vi "Windows Message Queue Example.vi"() -> ()   [LabVIEW 2017, in "Windows messages for Labview (32 and 64).lvlib"]
doc: "This VI demonstrates the use of the Windows Message Queue,\nwhich allows for VIs to be sensitized to specified Windows\nMessages so that they can programmatically respond to the\nmessage.\n\n The call to Create Windows Message Queue configures this VI\nto receive mouse move, left button down and right button down\nmessages. The Wait for Windows Messages waits for the next\nmessage asynchronously. Upon its receipt, it sends all messages\ncurrently in the queue to the case structure that processes them.\n\nIf the Wait times out, we also remove all messages from the\nqueue. This is to prevent messages from building up in the\nqueue when they are not immediately handled. It ensures that\nall messages are processed as soon as possible. \nIt also ensures that if no further messages are received, we still\nprocess the ones currently in the queue after timing out on \nthe Wait.\n\nIf the user clicks in \"Click here to Exit,\" the while loop exits and\nthe Windows message queue is destroyed."
uses:
  Windows messages for Labview (32 and 64).lvlib
  user32.dll
  shell32.dll
panel:
  out "output cluster":cluster{i16, i16}
  out "wParam":u64 format="%.0x"
  out "Files":string[](array[string])
  # "This VI demonstrates the use of the Windows Message Queue,\nwhich allows for VIs to be sensitized to specified Windows\nMessages so that they can programmatically respond to the\nmessage.\n\n The call to Create Windows Message Queue configures this VI\nto receive mouse move, left button down and right button down\nmessages.  The Wait for Windows Messages waits for the next\nmessage asynchronously.  Upon its receipt, it sends all messages\ncurrently in the queue to the case structure that processes them.\n\nIf the Wait times out, we also remove all messages from the\nqueue.  This is to prevent messages from building up in the\nqueue when they are not immediately handled.  It ensures that\nall messages are processed as soon as possible. \nIt also ensures that if no further messages are received, we still\nprocess the ones currently in the queue after timing out on \nthe Wait.\n\nIf the user clicks in \"Click here to Exit,\" the while loop exits and\nthe Windows message queue is destroyed."
  # "Bitmap picture"
  # "Value\tMeaning\nMK_CONTROL\n0x0008\nThe CTRL key is down.\nMK_LBUTTON\n0x0001\nThe left mouse button is down.\nMK_MBUTTON\n0x0010\nThe middle mouse button is down.\nMK_RBUTTON\n0x0002\nThe right mouse button is down.\nMK_SHIFT\n0x0004\nThe SHIFT key is down.\nMK_XBUTTON1\n0x0020\nThe first X button is down.\nMK_XBUTTON2\n0x0040\nThe second X button is down."
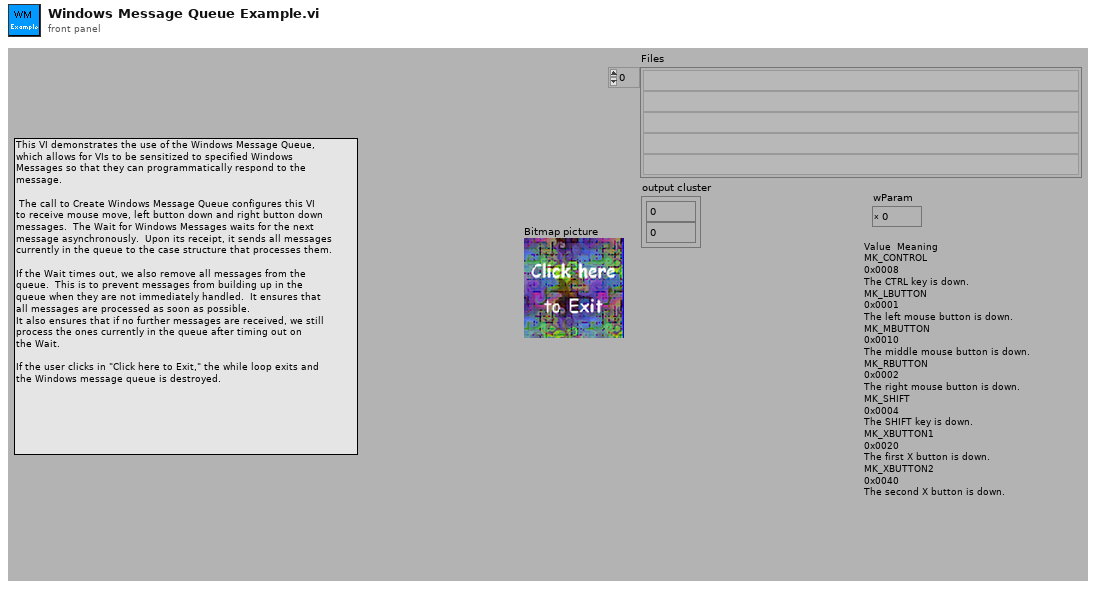
[diagram p1: front panel]
types:
  T1 = typedef "Windows messages for Labview (32 and 64).lvlib/Win Msg Queue RefNum.ctl" = refnum<k1>
  T2 = typedef "Windows messages for Labview (32 and 64).lvlib/windows message x64.ctl" = cluster{"hWnd":u64, "Msg":u32, "wParam":u64, "lParam":i32, "time":u32, "point":cluster{"X":i32, "Y":i32}}
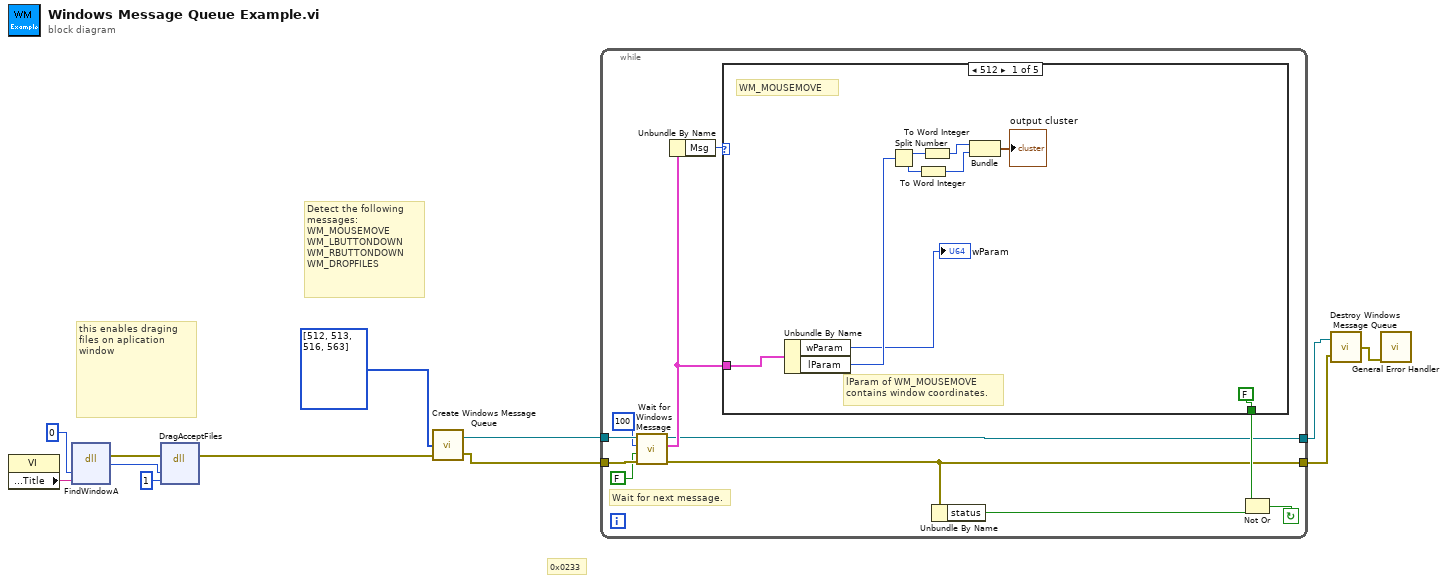
[diagram p0: block diagram]
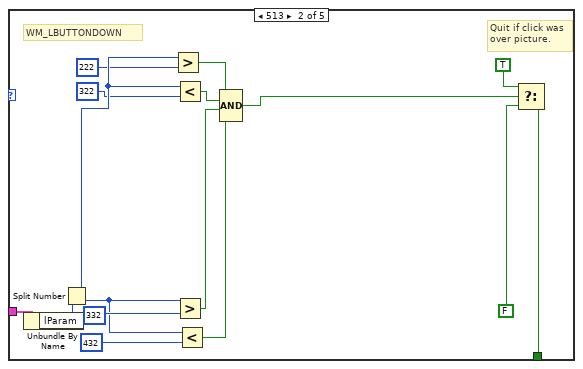
[diagram p2: hidden frame]
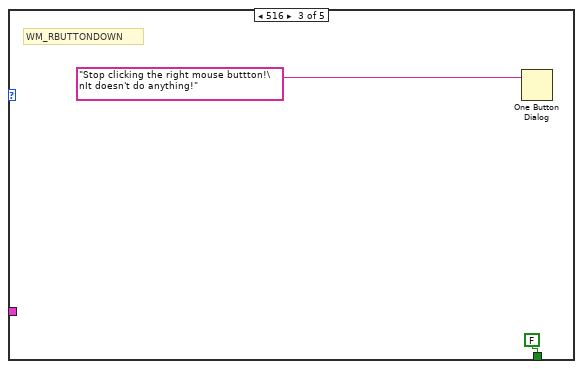
[diagram p3: hidden frame]
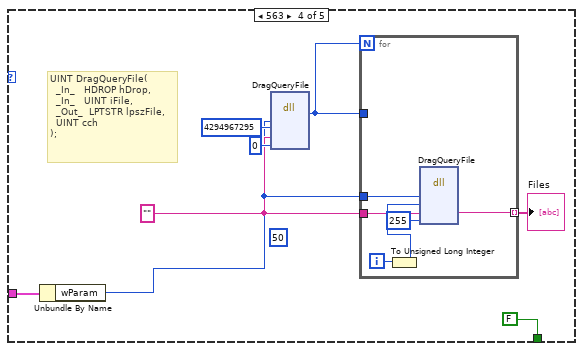
[diagram p4: hidden frame]
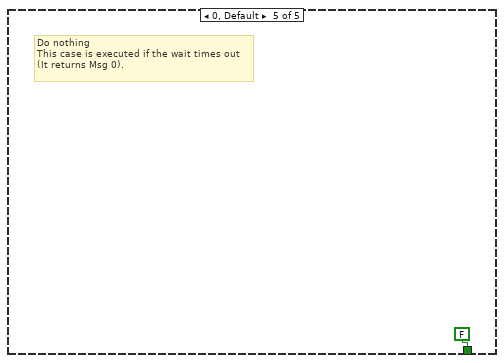
[diagram p5: hidden frame]
diagram:
  # "this enables draging files on aplication window"
  # "0x0233"
  # "Detect the following\nmessages:\nWM_MOUSEMOVE\nWM_LBUTTONDOWN\nWM_RBUTTONDOWN\nWM_DROPFILES"
  n1 = property class="VI"() -> ("Front Panel Window:Title"=w7:string)  [unwired: 2 in, 2 out]
  n2 = dll-call lib="user32.dll" fn="FindWindowA" label="FindWindow"("lpszClassName"=0, "lpszWindowName"=w7) -> (error out=w6:errorcluster, "hWnd"=w10:u32)  [unwired: 5 in, 1 out]
  n3 = dll-call lib="shell32.dll" fn="DragAcceptFiles"(error in=w6, "hWnd"=w10, "fAccept"=1) -> (error out=w11:errorcluster)  [unwired: 5 in, 1 out]
  n4 = call "Create Windows Message Queue.vi"("error in (no error)"=w11, "Messeges (none)"=u32[] [512, 513, 516, 563]) -> ("error out"=w4:errorcluster, "win msg queue"=w5:T1)  [unwired: 1 in]
  n5 = while {
    tunnel: [w14] -> w2
    tunnel: [w16] -> w3
    tunnel: w4 -> [w22]
    tunnel: w5 -> [w23]
    stop <- w21 continue-if-true
    # "Wait for next message."
    n6 = call "Wait for Windows Message.vi"("win msg queue"=w23, "ms timeout (-1)"=100, "ignore previous (F)"=FALSE ("ignore previous (T)"), "error in (no error)"=w22) -> ("win msg queue out"=w14:T1, "Message"=w15:T2, "error out"=w16:errorcluster)  [unwired: 3 out]
    n7 = Unbundle By Name(w15) -> ("Msg"=w13:u32)
    n8 = case shown="512" w13 {
      tunnel: [FALSE w35 FALSE FALSE FALSE] -> w18
      tunnel: w15 -> [w31 w34 _ w58 _]
      frame 512 {
        # "WM_MOUSEMOVE"
        # "lParam of WM_MOUSEMOVE\ncontains window coordinates."
        n9 = Unbundle By Name(w31) -> ("wParam"=→"wParam":u64, "lParam"=w30:i32)
        n10 = Split Number(x=w30) -> (hi(x)=w28:u16, lo(x)=w27:u16)
        n11 = To Word Integer(number=w27) -> (16bit integer=w25:i16)
        n12 = To Word Integer(number=w28) -> (16bit integer=w26:i16)
        n13 = Bundle(w26, w25) -> (→"output cluster":cluster{i16, i16})  [unwired: 1 in]
      }
      frame 513 {
        # "Quit if click was\nover picture."
        # "WM_LBUTTONDOWN"
        n14 = Unbundle By Name(w34) -> ("lParam"=w33:i32)
        n15 = Split Number(x=w33) -> (hi(x)=w45:u16, lo(x)=w47:u16)
        n16 = Greater?(x=w45, y=u16 222) -> (0:w42:bool)
        n17 = Less?(x=w45, y=u16 322) -> (x < y?=w41:bool)
        n18 = Greater?(x=w47, y=u16 332) -> (0:w40:bool)
        n19 = Less?(x=w47, y=u16 432) -> (x < y?=w39:bool)
        n20 = Compound Arithmetic op=AND(w42, w41, w40, w39) -> (w38:bool)
        n21 = Select(t=TRUE, s=w38, f=FALSE) -> (s? t:f=w35:bool)
      }
      frame 516 {
        # "WM_RBUTTONDOWN"
        n22 = One Button Dialog(message="Stop clicking the right mouse buttton!\nIt doesn't do anything!") -> ()  [unwired: 1 in, 1 out]
      }
      frame 563 {
        (unwired) 50
        w54 = ""
        # "UINT DragQueryFile(\n  _In_   HDROP hDrop,\n  _In_   UINT iFile,\n  _Out_  LPTSTR lpszFile,\n  UINT cch\n);"
        n23 = Unbundle By Name(w58) -> ("wParam"=w52:u64)
        n24 = dll-call lib="shell32.dll" fn="DragQueryFile"("hDrop"=w52, "iFile"=u32 4294967295, "lpszFile"=w54, "cch"=u32 0) -> ("out"=w53:u32)  [unwired: 7 in, 2 out]
        n25 = for {
          N: w53 -> [_]
          tunnel: w53 -> [_]
          tunnel: w54 -> [w64]
          tunnel: w52 -> [w60]
          tunnel: [w59] -> w51 mode=indexing
          i -> [w62]
          n26 = To Unsigned Long Integer(number=w62) -> (unsigned 32bit integer=w61:u32)
          n27 = dll-call lib="shell32.dll" fn="DragQueryFile"("hDrop"=w60, "iFile"=w61, "lpszFile"=w64, "cch"=u32 255) -> ("lpszFile"=w59:string)  [unwired: 7 in, 2 out]
        }
        "Files" <- w51
      }
      frame 0, Default {
        # "Do nothing\nThis case is executed if the wait times out\n(It returns Msg 0)."
      }
    }
    n28 = Unbundle By Name(w16) -> ("status"=w17:bool)
    n29 = Not Or(1:w17, 2:w18) -> (0:w21:bool)
  }
  n30 = call "Destroy Windows Message Queue.vi"("error in (no error)"=w3, "win msg queue"=w2) -> ("error out"=w1:errorcluster)
  n31 = call <vilib>:"General Error Handler.vi"("error in (no error)"=w1) -> ()  [unwired: 10 in, 5 out]
